vi "RelativePositionCombined2_KCubeDCServo.vi"(8 "element 2":dbl, 9 "element 1":dbl, 10 "device 2":refnum<k24>, 11 "device 1":refnum<k24>) -> ()   [LabVIEW 2019]
doc: "relative position given a value. used for direct inputting of relative position value"
uses:
  D:/Victor Sun/optical trap control/Kinesis/ThorLabs.MotionControl.KCube.DCServoCLI.dll
  Kinesis/ThorLabs.MotionControl.KCube.DCServoCLI.dll
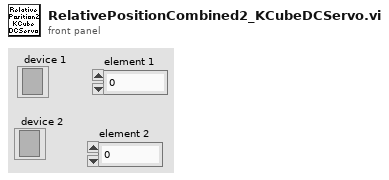
[diagram p1: front panel]
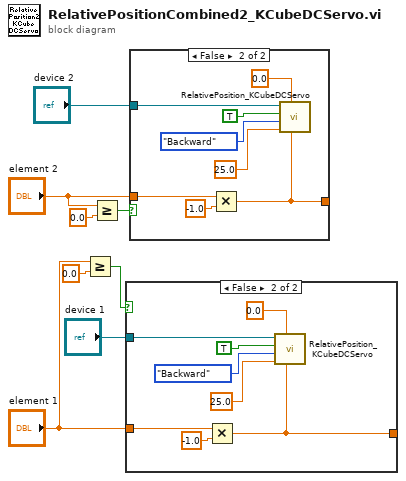
[diagram p0: block diagram]
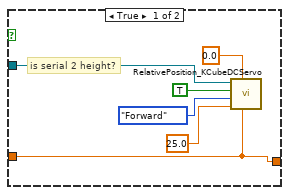
[diagram p2: hidden frame]
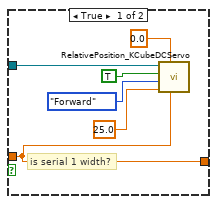
[diagram p3: hidden frame]
diagram:
  n1 = Greater Or Equal?(x="element 1", y=0.0) -> (x >= y?=w5:bool)
  n2 = Greater Or Equal?(x="element 2", y=0.0) -> (x >= y?=w2:bool)
  n3 = case shown="False" w5 {
    tunnel: "element 1" -> [w10 w21]
    tunnel: "device 1" -> [w9 w20]
    tunnel: [w10 w17] -> _
    frame True {
      # "is serial 2 height?"
      n4 = call "RelativePosition_KCubeDCServo.vi"("set jog step size"=w10, "lower limit"=0.0, "upper limit"=25.0, "Direction Control"=enum16{"Backward", "Forward"}."Forward", "direction button"=TRUE, ".NET Refnum in"=w9) -> ()  [unwired: 4 in, 2 out]
    }
    frame False {
      n5 = Multiply(x=w21, y=-1.0) -> (x*y=w17:dbl)
      n6 = call "RelativePosition_KCubeDCServo.vi"("set jog step size"=w17, "lower limit"=0.0, "upper limit"=25.0, "Direction Control"=enum16{"Backward", "Forward"}."Backward", "direction button"=TRUE, ".NET Refnum in"=w20) -> ()  [unwired: 4 in, 2 out]
    }
  }
  n7 = case shown="False" w2 {
    tunnel: "element 2" -> [w24 w31]
    tunnel: "device 2" -> [w23 w29]
    tunnel: [w24 w30] -> _
    frame True {
      # "is serial 1 width?"
      n8 = call "RelativePosition_KCubeDCServo.vi"("set jog step size"=w24, "lower limit"=0.0, "upper limit"=25.0, "Direction Control"=enum16{"Backward", "Forward"}."Forward", "direction button"=TRUE, ".NET Refnum in"=w23) -> ()  [unwired: 4 in, 2 out]
    }
    frame False {
      n9 = Multiply(x=w31, y=-1.0) -> (x*y=w30:dbl)
      n10 = call "RelativePosition_KCubeDCServo.vi"("set jog step size"=w30, "lower limit"=0.0, "upper limit"=25.0, "Direction Control"=enum16{"Backward", "Forward"}."Backward", "direction button"=TRUE, ".NET Refnum in"=w29) -> ()  [unwired: 4 in, 2 out]
    }
  }
